vi "colorToRGB.vi"(11 "color":u32) -> (1 "upper limit":u8, 2 "upper limit 3":u8, 3 "upper limit 2":u8)   [LabVIEW 2014]
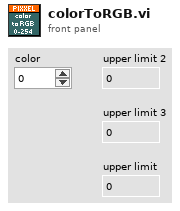
[diagram p1: front panel]
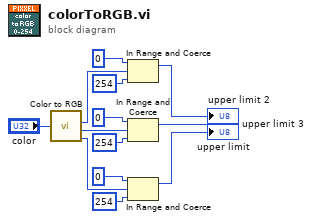
[diagram p0: block diagram]
diagram:
  n1 = call <vilib>:"Color to RGB.vi"("Color"="color") -> ("R"=w1:u8, "G"=w2:u8, "B"=w10:u8)  [unwired: 1 out]
  n2 = In Range and Coerce(upper limit=u8 0, x=w1, lower limit=u8 254) -> (coerced(x)=→"upper limit 2":u8)  [unwired: 1 out]
  n3 = In Range and Coerce(upper limit=u8 0, x=w2, lower limit=u8 254) -> (coerced(x)=→"upper limit 3":u8)  [unwired: 1 out]
  n4 = In Range and Coerce(upper limit=u8 0, x=w10, lower limit=u8 254) -> (coerced(x)=→"upper limit":u8)  [unwired: 1 out]
